vi "files_to_sent.vi"(6 "pattern":string="*.tdms", 7 "Directory":path) -> (0 "error IO":errorcluster, 1 "file_1 path":path caption="Первый", 2 "names":string[](array[string]) caption="Список необработанных", 3 "directory dup":path)   [LabVIEW 2010]
panel:
  out "y":i32
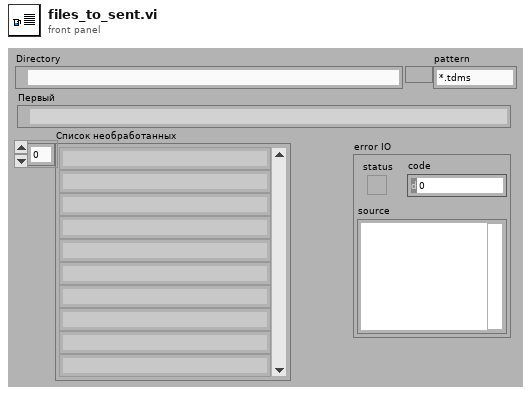
[diagram p1: front panel]
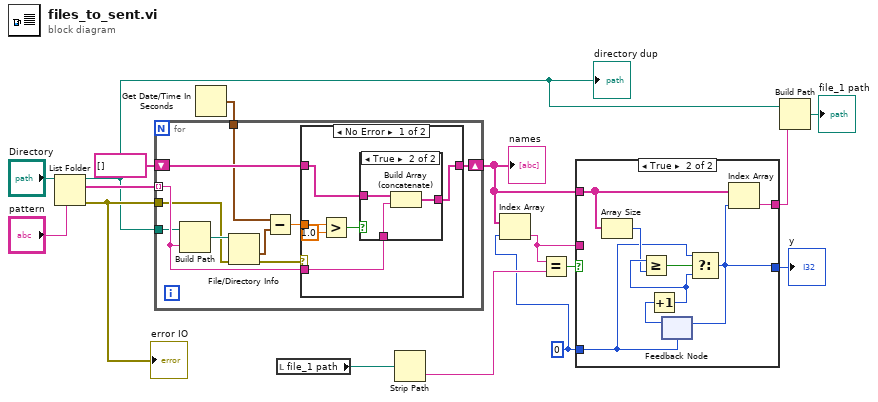
[diagram p0: block diagram]
diagram:
  w2 = 0 ("y")
  n1 = List Folder(path="Directory", pattern="pattern") -> (path out=w11:path, filenames=w15:string[], error out=w13:errorcluster)  [unwired: 2 in, 1 out]
  "directory dup" <- w11
  "error IO" <- w13
  n2 = Get Date/Time In Seconds() -> (seconds since 1Jan1904=w3:timestamp)
  n3 = for {
    tunnel: w15 -> [w24] mode=indexing
    shift-right: [w26] -> w7
    shift-left: string[] [] -> [w25]
    tunnel: w13 -> [w18]
    tunnel: w11 -> [w23]
    tunnel: w3 -> [w17]
    n4 = Build Path(base path=w23, name or relative path=w24) -> (appended path=w22:path)
    n5 = File/Directory Info(path=w22, error in=w18) -> (last mod=w20:timestamp, error out=w21:errorcluster)  [unwired: 5 out]
    n6 = Subtract(x=w17, y=w20) -> (x-y=w19:dbl)
    n7 = case shown="No Error" w21 {
      tunnel: w24 -> [w32 _]
      tunnel: [w31 w37] -> w26
      tunnel: w25 -> [w30 w37]
      tunnel: w19 -> [w29 _]
      frame No Error {
        n8 = Greater?(x=w29, y=1.0) -> (0:w28:bool)
        n9 = case shown="True" w28 {
          tunnel: w32 -> [_ w36]
          tunnel: [w33 w35] -> w31
          tunnel: w30 -> [w33 w34]
          frame False {
          }
          frame True {
            n10 = Build Array (concatenate)(w34, w36) -> (w35:string[])
          }
        }
      }
      frame Error {
      }
    }
  }
  "names" <- w7
  n11 = local read "file_1 path"() -> (w10:path)
  n12 = Strip Path(path=w10) -> (name=w9:string)  [unwired: 1 out]
  n13 = Index Array(array=w7, index=w2) -> (element=w5:string)
  n14 = Equal?(x=w5, y=w9) -> (x = y?=w8:bool)
  n15 = case shown="True" w8 {
    tunnel: w7 -> [_ w46]
    tunnel: [w39 w42] -> w4
    tunnel: w5 -> [w39 _]
    tunnel: w2 -> [w38 w41]
    tunnel: [w38 w40] -> w1
    frame False {
    }
    frame True {
      n16 = Array Size(array=w46) -> (size(s)=w44:i32)
      n17 = feedback #1(w41) -> (w47:i32)
      n18 = Increment(x=w47) -> (x+1=w45:i32)
      n19 = Greater Or Equal?(x=w45, y=w44) -> (x >= y?=w43:bool)
      n20 = Select(t=w41, s=w43, f=w45) -> (s? t:f=w40:i32)
      n21 = feedback-in #1(w40) -> ()
      n22 = Index Array(array=w46, index=w40) -> (element=w42:string)
    }
  }
  "y" <- w1
  n23 = Build Path(base path=w11, name or relative path=w4) -> (appended path=→"file_1 path":path)
